vi "mnist Keras.vi"() -> ()   [LabVIEW 2020]
panel:
  out "is_draw":bool
  in  "Train":bool
  out "draw timestamp":u32
  out "Status":string
  out "Predictions":sgl[](array[slide]) scale=0.0..1.0
  in  "Clear":bool
  out "Prediction":sgl
  out "Predicted Label":i32
  out "Training Results : Loss, Accuracy":dbl[](array[numeric])
  in  "Epochs":i32=3
  in  "Metrics":string="accuracy"
  in  "Loss":string="sparse_categorical_crossentropy"
  in  "Optimizer":string="adam"
  in  "stop":bool
  out "Draw pane":picture
  # "Overview: This example shows how to use the deep learning API to perform numeric classification using the Python Keras library. The model is of sequential type and is compiled using the optimizer provided by Keras. Trained using the mnist dataset, this model recognizes and classifies numbers you draw on the front panel.\nRequirements: Python 3.6 (64-bits)\nInstructions:\n1. Make sure you have TensorFlow and Keras installed in your Python environment.\n2. Open mnist Keras.vi.\n3. Run the VI. After the model has been compiled and trained, the Status indicator changes to \"Model_Predicting\".\n4. Drag the mouse into the draw pane to draw a number and the model will output the prediction."
  # "0\n1\n2\n3\n4\n5\n6\n7\n8\n9"
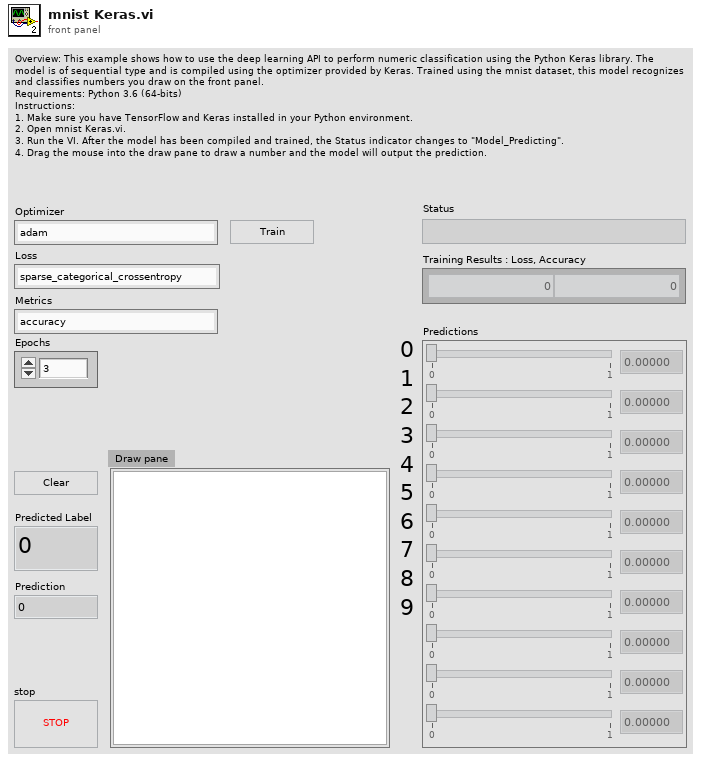
[diagram p1: front panel]
types:
  T1 = cluster{"Width":u16, "Style":enum32{"Solid", "Dash", "Dot", "DashDot", "DashDotDot"}}
  T2 = typedef "LVMouseTypeDef.ctl" = cluster{"Mouse Position":cluster{"X":i32, "Y":i32}, "Mouse Modifiers":cluster{"Button Down":bool, "Shift Mod":bool, "Menu Mod":bool, "Option Mod":bool}}
  T3 = cluster{"Button Down":bool, "Shift Mod":bool, "Menu Mod":bool, "Option Mod":bool}
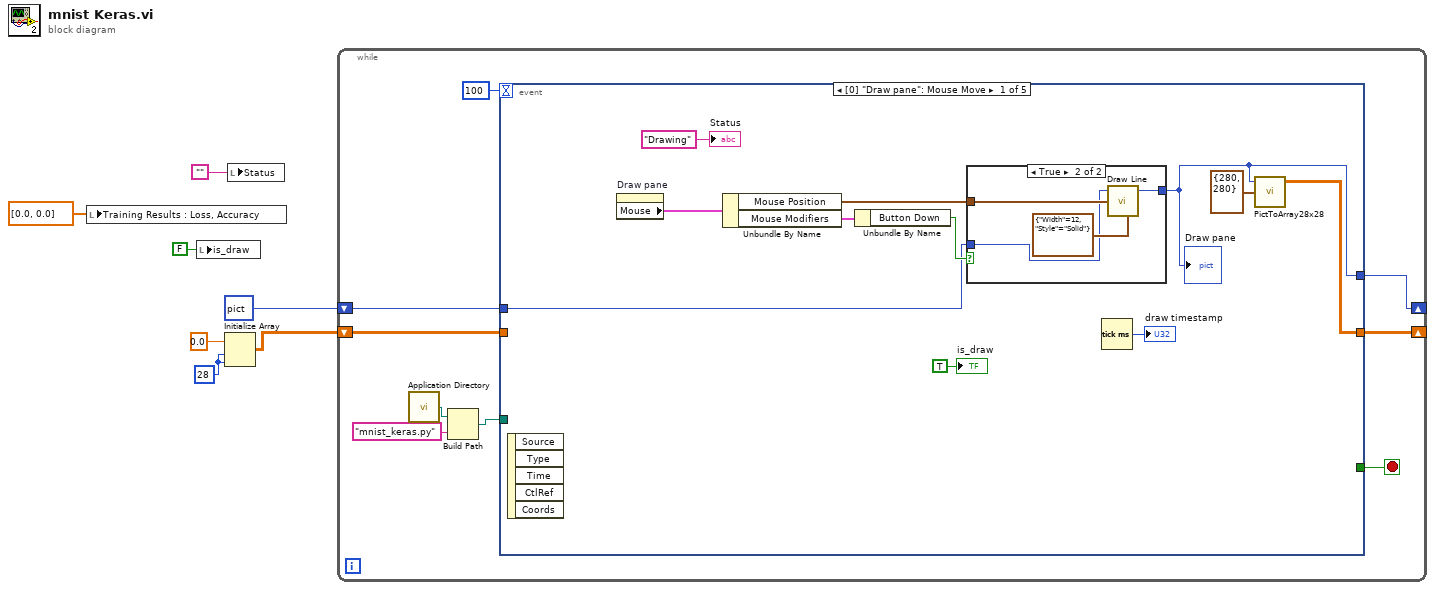
[diagram p0: block diagram]
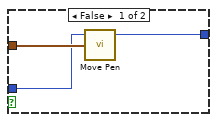
[diagram p2: hidden frame]
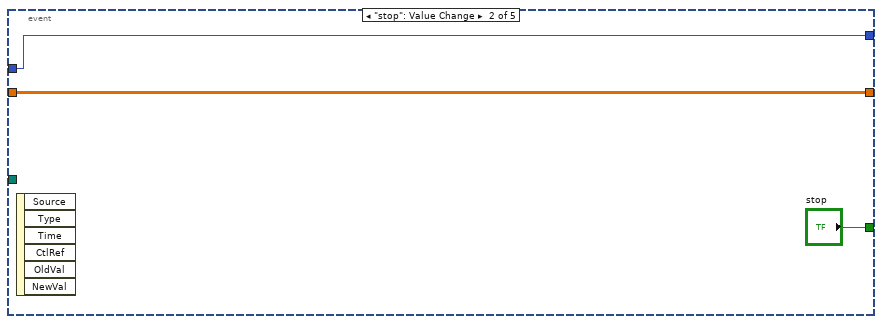
[diagram p3: hidden frame]
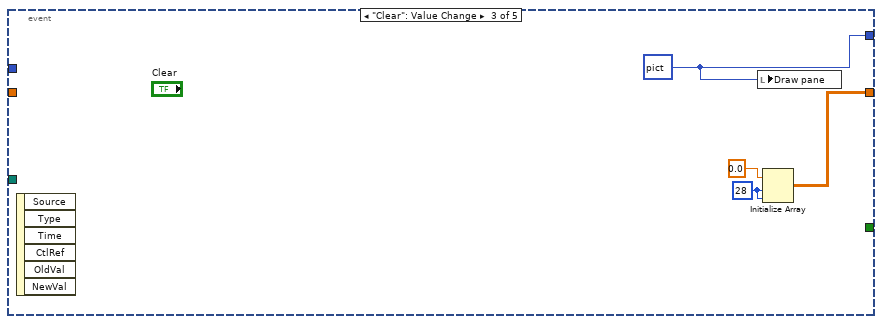
[diagram p4: hidden frame]
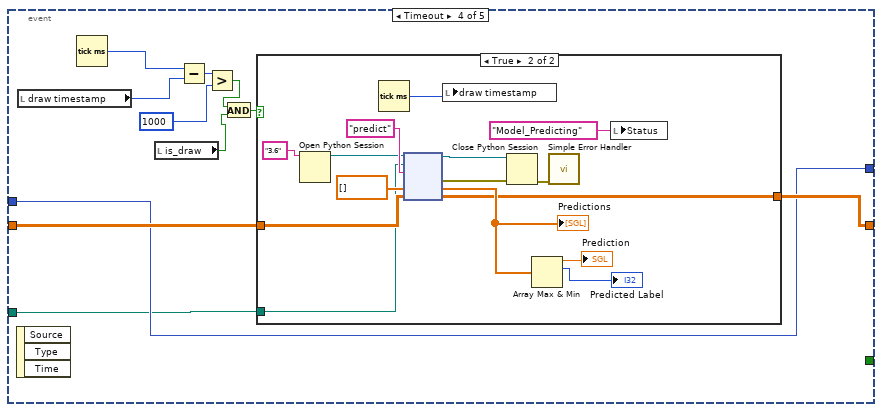
[diagram p5: hidden frame]
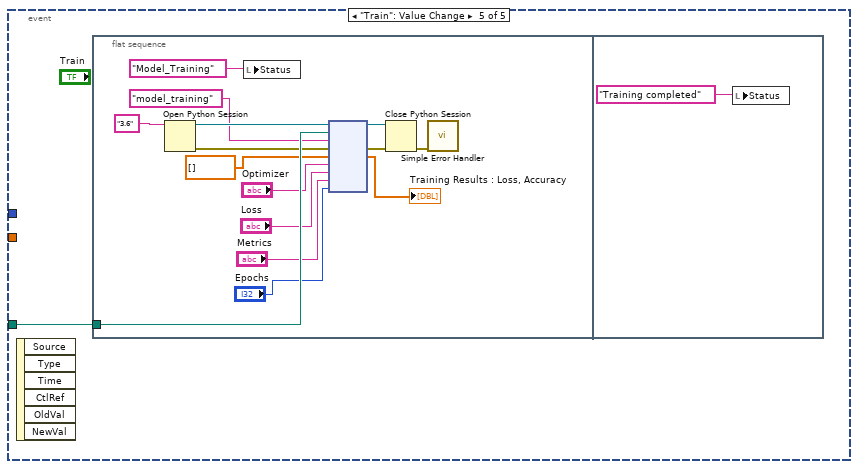
[diagram p7: hidden frame]
diagram:
  w5 = 28 ("dimension size")
  n1 = local write "Training Results : Loss, Accuracy"(dbl[] [0.0, 0.0] ("Training Results : Loss, Accuracy")) -> ()
  n2 = local write "is_draw"(FALSE ("is_draw")) -> ()
  n3 = Initialize Array(sgl 0.0 ("element"), w5, w5) -> (w4:sgl[][])
  n4 = local write "Status"("") -> ()
  n5 = while {
    shift-right: [w16] -> _
    shift-left: picture data[5B] ("empty picture") -> [w15]
    shift-right: [w12] -> _
    shift-left: w4 -> [w11]
    stop <- w14 stop-if-true
    n6 = call <vilib>:"Application Directory.vi"() -> ("Application Directory"=w9:path)
    n7 = Build Path(base path=w9, name or relative path="mnist_keras.py") -> (appended path=w8:path)
    n8 = event shown="[0] \"Draw pane\": Mouse Move" {
      selector: _ -> [_ _ _ _ _]
      dyn-events: _ -> [_ _ _ _ _]
      timeout: 100 -> [_ _ _ _ _]
      tunnel: [w20 w36 w38 w50 _] -> w16
      tunnel: w15 -> [w23 w36 _ w50 _]
      tunnel: [_ "stop" _ _ _] -> w14
      tunnel: [w19 w35 w40 w51 _] -> w12
      tunnel: w11 -> [_ w35 _ w52 _]
      tunnel: w8 -> [_ _ _ w49 w69]
      event "Draw pane": Mouse Move {
        n9 = event-data() -> ()  [unwired: 1 in, 5 out]
        n10 = property on="Draw pane" class="Pict"() -> ("Mouse"=w27:T2)  [unwired: 2 in, 2 out]
        n11 = Unbundle By Name(w27) -> ("Mouse Position"=w25:cluster{"X":i32, "Y":i32}, "Mouse Modifiers"=w26:T3)
        n12 = Unbundle By Name(w26) -> ("Button Down"=w24:bool)
        n13 = case shown="True" w24 {
          tunnel: w25 -> [w29 w34]
          tunnel: [w30 w33] -> w20
          tunnel: w23 -> [w28 w31]
          frame False {
            n14 = call <vilib>:"Move Pen.vi"("new position"=w29, "picture"=w28) -> ("new picture"=w30:picture)  [unwired: 3 in]
          }
          frame True {
            n15 = call <vilib>:"Draw Line.vi"("picture"=w31, "end point"=w34, "pen"=T1 {"Width"=12, "Style"=enum."Solid"}) -> ("new picture"=w33:picture)  [unwired: 6 in]
          }
        }
        "Draw pane" <- w20
        n16 = Tick Count (ms)() -> (millisecond timer value=→"draw timestamp":u32)
        n17 = call "PictToArray28x28.vi"("Draw Area Size"=cluster{"Width":u32, "Height":u32} {"Width"=280, "Height"=280}, "Picture"=w20) -> ("Array"=w19:dbl[][])  [unwired: 1 in, 2 out]
        "Status" <- "Drawing" ("Status")
        "is_draw" <- TRUE ("is_draw")
      }
      event "stop": Value Change {
        n18 = event-data() -> ()  [unwired: 1 in, 6 out]
      }
      event "Clear": Value Change {
        w39 = 28 ("dimension size")
        w38 = picture data[5B] ("empty picture")
        n19 = event-data() -> ()  [unwired: 1 in, 6 out]
        n20 = local write "Draw pane"(w38) -> ()
        n21 = Initialize Array(sgl 0.0 ("element"), w39, w39) -> (w40:sgl[][])
      }
      event Timeout {
        n22 = event-data() -> ()  [unwired: 1 in, 3 out]
        n23 = local read "draw timestamp"() -> (w47:u32)
        n24 = Tick Count (ms)() -> (millisecond timer value=w48:u32)
        n25 = local read "is_draw"() -> (w42:bool)
        n26 = Subtract(x=w48, y=w47) -> (x-y=w46:u32)
        n27 = Greater?(x=w46, y=u32 1000) -> (0:w44:bool)
        n28 = And(x=w44, y=w42) -> (x .and. y?=w43:bool)
        n29 = case shown="True" w43 {
          tunnel: w52 -> [w53 w63]
          tunnel: [w53 w62] -> w51
          tunnel: w49 -> [_ w60]
          frame False {
          }
          frame True {
            n30 = Open Python Session(python version="3.6") -> (session out=w54:refnum<k35>)  [unwired: 2 in, 1 out]
            n31 = Tick Count (ms)() -> (millisecond timer value=w59:u32)
            n32 = node(w54, w60, "predict" ("함수 이름"), sgl[] [], w63) -> (w57:refnum<k35>, w56:errorcluster, w66:sgl[], w62:dbl[][])  [unwired: 1 in, 2 out]
            "Predictions" <- w66
            n33 = local write "draw timestamp"(w59) -> ()
            n34 = Close Python Session(session in=w57, error in=w56) -> (11:w58:errorcluster)
            n35 = Array Max & Min(array=w66) -> (max value=→"Prediction":sgl, max index (indices)=→"Predicted Label":i32)  [unwired: 2 out]
            n36 = call <vilib>:"Simple Error Handler.vi"("error in (no error)"=w58) -> ()  [unwired: 4 in, 5 out]
            n37 = local write "Status"("Model_Predicting" ("Status")) -> ()
          }
        }
      }
      event "Train": Value Change {
        n38 = event-data() -> ()  [unwired: 1 in, 6 out]
        n39 = flat-sequence {
          tunnel: w69 -> [w84]
          frame #0 {
            n40 = Open Python Session(python version="3.6") -> (session out=w77:refnum<k35>, error out=w78:errorcluster)  [unwired: 2 in]
            n41 = local write "Status"("Model_Training" ("Status")) -> ()
            n42 = node(w77, w84, "model_training" ("함수 이름"), w78, dbl[] [], "Optimizer", "Loss", "Metrics", "Epochs") -> (w72:refnum<k35>, w71:errorcluster, →"Training Results : Loss, Accuracy":dbl[])  [unwired: 4 in, 2 out]
            n43 = Close Python Session(session in=w72, error in=w71) -> (11:w73:errorcluster)
            n44 = call <vilib>:"Simple Error Handler.vi"("error in (no error)"=w73) -> ()  [unwired: 4 in, 5 out]
          }
          frame #1 {
            n45 = local write "Status"("Training completed" ("Status")) -> ()
          }
        }
      }
    }
  }
